vi "example_get_device_status.vi"() -> ()   [LabVIEW 2012]
doc: "EXAMPLE: Get Device Status\n\nThis example VI demonstrates how to retrieve the current status value(s) of the referenced device. There are two types of states the device can be in. One is a motion based state, where the device can be in only one of these states:\n\n(1) Idle (IDLE)\n(2) Running at constant speed (CONST)\n(3) Accelerating (ACCEL)\n(4) Decelerating (DECEL)\n\nThe other is non-motion based, where multiple states can exist at one time (in addition to the single motion state above)\n\nNOTE: if any of the following states exist in the \"other_states\" array output, then they are considered logically TRUE\n\n(1) Home input switch status (HOME_SWITCH)\n(2) Minus limit input switch status (-LIMIT_SWITCH)\n(3) Plus limit input switch status (+LIMIT_SWITCH)\n(4) Minus limit error (-LIMIT_ERR)\n(5) Plus limit error (+LIMIT_ERR)\n(6) Communication timeout counter alarm (COMM_ERR)\n\nProduced By:\n\nChristopher Lemieux\nKod Integrations, LLC\n4835 Marianne Drive\nMount Airy, MD 21771\nhttp://www.kodintegrations.com\nemail: clemieux@kodintegrations.com\nphone: (240) 687-1288"
uses:
  utilities/getters/controls/status_states.ctl
panel:
  out "other_states":T1[](array[typedef])
  out "motion_state":T1=enum."CONST"
  in  "device_index (def=0)":i32
  out "error out":errorcluster
  in  "error in (no error)":errorcluster
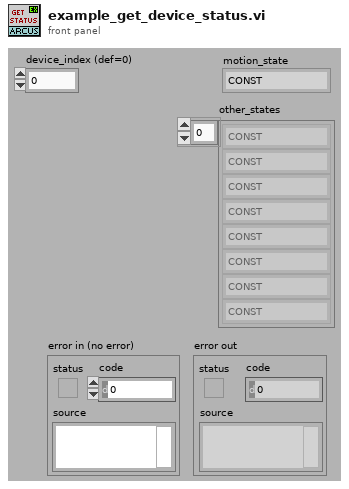
[diagram p1: front panel]
types:
  T1 = typedef "status_states.ctl" = enum16{"IDLE", "CONST", "ACCEL", "DECEL", "HOME_SWITCH", "-LIMIT_SWITCH", "+LIMIT_SWITCH", "-LIMIT_ERR", "+LIMIT_ERR", "COMM_ERR"}
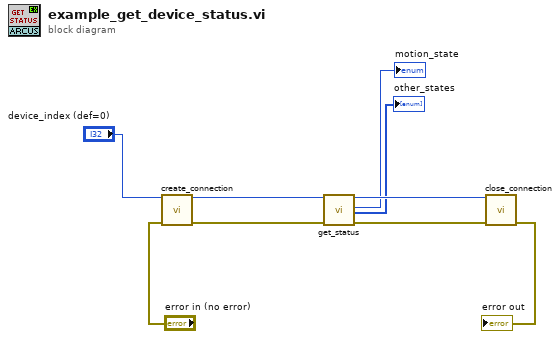
[diagram p0: block diagram]
diagram:
  n1 = call "create_connection.vi"("device_index (def=0)"="device_index (def=0)", "error in (no error)"="error in (no error)") -> ("reference"=w5:i32, "error out"=w6:errorcluster)  [unwired: 12 in]
  n2 = call "get_status.vi"("reference (in)"=w5, "error in (no error)"=w6) -> ("reference (dup)"=w4:i32, "motion_state"=→"motion_state":T1, "other_states"=→"other_states":T1[], "error out"=w3:errorcluster)  [unwired: 13 in, 1 out]
  n3 = call "close_connection.vi"("reference"=w4, "error in (no error)"=w3) -> ("error out"=→"error out":errorcluster)  [unwired: 13 in]
